vi "GyroTest.vi"() -> ()   [LabVIEW 2016]
uses:
  Gyro/GyroErrorCodes.ctl
  Telemetry/TelemetryFields.ctl
  <vilib>/rvi/Emulation/niFpgaGetClockAttributes.vi
  <vilib>/rvi/Emulation/niFpgaSctlEmulationGetInTimedLoop.vi
  <vilib>/rvi/Emulation/niFpgaEmulationReportErrorSimple.vi
  <vilib>/rvi/Emulation/niFpgaEmulationIsFPGAContextNoSignature.vi
  <vilib>/rvi/errors/niFpgaSetErrorForExecOnDevCompSimple.vi
  <vilib>/rvi/eio/common/nirviEmuReportErrorAndStop.vi
  <vilib>/rvi/DataTransferAndStorage/Container/Common/niFpgaContainerGetUniqueNameForEmu.vi
  <vilib>/rvi/FIFO/Fifo_Resource/nirvififoEmulationSetSize.vi
  <vilib>/rvi/FIFO/Fifo_Resource/nirviFifoEmulationQueueMgr.vi
  <instcachedir>/0/nirviFifoEmulationQueueMgr_E5CAEC123FF24DC58D834DCA3CDAA9B5.lvgen/nirviFifoEmulationQueueMgr_E5CAEC123FF24DC58D834DCA3CDAA9B5_004.vi
  <vilib>/Utility/error.llb/Clear Errors.vi
  <vilib>/rvi/FIFO/Fifo_Resource/nirvififoEmulationCreateLock.vi
  <vilib>/rvi/Emulation/niFpgaProcessEmulError.vi
  <vilib>/rvi/FIFO/Fifo_Resource/nirvififoEmulationObtainLock.vi
  <vilib>/rvi/FIFO/Fifo_Resource/nirvififoEmulationReleaseLock.vi
  <vilib>/rvi/occurrence/nirviWaitOnOccurrenceBase.vi
  <vilib>/rvi/errors/nirviReportUnexpectedCaseInternalError.vi
  <vilib>/rvi/errors/nirviReportUnexpectedCaseInternalError (U32).vi
  <vilib>/rvi/FIFO/Fifo_Resource/nirvififoEmulationDetermineInputValidOut.vi
  <vilib>/rvi/Emulation/niFpgaCriticalErrorInLSC.vi
  <instcachedir>/0/nirviFifoEmulationQueueMgr_E5CAEC123FF24DC58D834DCA3CDAA9B5.lvgen/nirviFifoEmulationQueueMgr_E5CAEC123FF24DC58D834DCA3CDAA9B5_028.vi
  <instcachedir>/0/nirviFifoEmulationQueueMgr_E5CAEC123FF24DC58D834DCA3CDAA9B5.lvgen/nirviFifoEmulationQueueMgr_E5CAEC123FF24DC58D834DCA3CDAA9B5_029.vi
  <instcachedir>/0/nirviFifoEmulationQueueMgr_E5CAEC123FF24DC58D834DCA3CDAA9B5.lvgen/nirviFifoEmulationQueueMgr_E5CAEC123FF24DC58D834DCA3CDAA9B5_039.vi
  <instcachedir>/0/nirviFifoEmulationQueueMgr_E5CAEC123FF24DC58D834DCA3CDAA9B5.lvgen/nirviFifoEmulationQueueMgr_E5CAEC123FF24DC58D834DCA3CDAA9B5_038.vi
  <instcachedir>/0/nirviFifoEmulationQueueMgr_E5CAEC123FF24DC58D834DCA3CDAA9B5.lvgen/nirviFifoEmulationQueueMgr_E5CAEC123FF24DC58D834DCA3CDAA9B5_035.vi
  <instcachedir>/0/nirviFifoEmulationQueueMgr_E5CAEC123FF24DC58D834DCA3CDAA9B5.lvgen/nirviFifoEmulationQueueMgr_E5CAEC123FF24DC58D834DCA3CDAA9B5_033.vi
  <instcachedir>/0/nirviFifoEmulationQueueMgr_E5CAEC123FF24DC58D834DCA3CDAA9B5.lvgen/nirviFifoEmulationQueueMgr_E5CAEC123FF24DC58D834DCA3CDAA9B5_009.vi
  <instcachedir>/0/nirviFifoEmulationQueueMgr_E5CAEC123FF24DC58D834DCA3CDAA9B5.lvgen/nirviFifoEmulationQueueMgr_E5CAEC123FF24DC58D834DCA3CDAA9B5_026.vi
  <vilib>/rvi/DataTransferAndStorage/Container/XNode/niFpgaContainer.xnode
  <vilib>/rvi/FIFO/Fifo_Resource/nirvififoEmulationRead.vi
  <vilib>/rvi/FIFO/Fifo_Resource/nirvififoEmulationWrite.vi
panel:
  out "GyroErrorCodeTimestamp":u64
  out "GyroErrorCode":T1
  out "GyroSampleTimestamp":u64
  out "GyroRxFrames":u64
  out "GyroTxFrames":u64
  out "GyroRxBytes":u64
  out "GyroTxBytes":u64
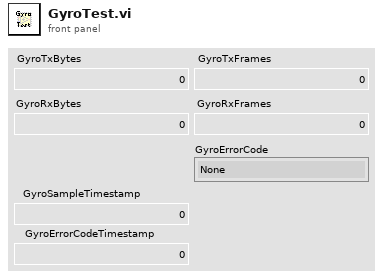
[diagram p1: front panel]
types:
  T1 = typedef "GyroErrorCodes.ctl" = enum8{"None", "ResponseHeaderError", "ResponseCRCError", "ResponseTimeoutError", "ResponseChecksumError"}
  T2 = cluster{"Timestamp":u64, "Accelerometer1Voltage":sgl, "Accelerometer2Voltage":sgl, "Accelerometer3Voltage":sgl, "Accelerometer4Voltage":sgl, "Accelerometer5Voltage":sgl, "Accelerometer6Voltage":sgl, "Accelerometer7Voltage":sgl, "Accelerometer8Voltage":sgl, "Accelerometer1Acceleration":sgl, "Accelerometer2Acceleration":sgl, "Accelerometer3Acceleration":sgl, "Accelerometer4Acceleration":sgl, "Accelerometer5Acceleration":sgl, "Accelerometer6Acceleration":sgl, "Accelerometer7Acceleration":sgl, "Accelerometer8Acceleration":sgl, "AngularAccelerationX":sgl, "AngularAccelerationY":sgl, "AngularAccelerationZ":sgl}
  T3 = cluster{"Timestamp":u64, "TxBytes":u64, "RxBytes":u64, "TxFrames":u64, "RxFrames":u64, "ErrorCode":enum8{"None", "ResponseAddressError", "ResponseFunctionCodeError", "ResponseByteCountError", "ResponseCRCError", "ResponseUnknownError", "ResponseTimeoutError", "SensorReportsIllegalFunction", "SensorReportsIllegalDataAddress"}}
  T4 = cluster{"Timestamp":u64, "TxBytes":u64, "RxBytes":u64, "TxFrames":u64, "RxFrames":u64, "RawAngle":i32, "ZenithAngle":sgl}
  T5 = cluster{"Timestamp":u64, "TxBytes":u64, "RxBytes":u64, "TxFrames":u64, "RxFrames":u64, "ErrorCode":enum16{"None", "ResponseUnknownError", "ResponseInvalidError", "ResponseTimeoutError", "SensorIndicatesInvalidCommandError", "SensorIndicatesCommunicationTimeoutError", "SensorIndicatesDataLengthError", "SensorIndicatesNumberOfParametersError", "SensorIndicatesParameterError", "SensorIndicatesCommunicationError", "SensorIndicatesIDNumberError", "SensorIndicatesExpansionLineError", "SensorIndicatesWriteControlError"}}
  T6 = cluster{"Timestamp":u64, "TxBytes":u64, "RxBytes":u64, "TxFrames":u64, "RxFrames":u64, "Sensor1Raw":i32, "Sensor2Raw":i32, "Sensor3Raw":i32, "Sensor4Raw":i32, "Sensor5Raw":i32, "Sensor6Raw":i32, "Sensor7Raw":i32, "Sensor8Raw":i32, "Sensor1Eng":sgl, "Sensor2Eng":sgl, "Sensor3Eng":sgl, "Sensor4Eng":sgl, "Sensor5Eng":sgl, "Sensor6Eng":sgl, "Sensor7Eng":sgl, "Sensor8Eng":sgl, "PositionX":sgl, "PositionY":sgl, "PositionZ":sgl, "RotationX":sgl, "RotationY":sgl, "RotationZ":sgl}
  T7 = typedef "TelemetryFields.ctl" = enum16{"None", "InclinometerTxBytes", "InclinometerRxBytes", "InclinometerTxFrames", "InclinometerRxFrames", "InclinometerErrorTimestamp", "InclinometerErrorCode", "InclinometerSampleTimestamp", "InclinometerRawAngle", "InclinometerZenithAngle", "DisplacementTxBytes", "DisplacementRxBytes", "DisplacementTxFrames", "DisplacementRxFrames", "DisplacementErrorTimestamp", "DisplacementErrorCode", "DisplacementSampleTimestamp", "DisplacementRaw1", "DisplacementRaw2", "DisplacementRaw3", "DisplacementRaw4", "DisplacementRaw5", "DisplacementRaw6", "DisplacementRaw7", "DisplacementRaw8", "DisplacementEng1", "DisplacementEng2", "DisplacementEng3", "DisplacementEng4", "DisplacementEng5", "DisplacementEng6", "DisplacementEng7", "DisplacementEng8", "DisplacementPositionX", "DisplacementPositionY", "DisplacementPositionZ", "DisplacementRotationX", "DisplacementRotationY", "DisplacementRotationZ", "AccelerometerSampleCount", "AccelerometerSampleTimestamp", "AccelerometerRaw1", "AccelerometerRaw2", "AccelerometerRaw3", "AccelerometerRaw4", "AccelerometerRaw5", "AccelerometerRaw6", "AccelerometerRaw7", "AccelerometerRaw8", "AccelerometerEng1", "AccelerometerEng2", "AccelerometerEng3", "AccelerometerEng4", "AccelerometerEng5", "AccelerometerEng6", "AccelerometerEng7", "AccelerometerEng8", "AngularAccelerationX", "AngularAccelerationY", "AngularAccelerationZ", "GyroTxBytes", "GyroRxBytes", "GyroTxFrames", "GyroRxFrames", "GyroErrorTimestamp", "GyroErrorCode", "GyroSampleTimestamp", "AngularVelocityX", "AngularVelocityY", "AngularVelocityZ", "GyroStatus", "GyroSequenceNumber", "GyroTemperature", "GyroBITTimestamp", "GyroBIT0", "GyroBIT1", "GyroBIT2", "GyroBIT3", "GyroBIT4", "GyroBIT5", "GyroBIT6", "GyroBIT7"}
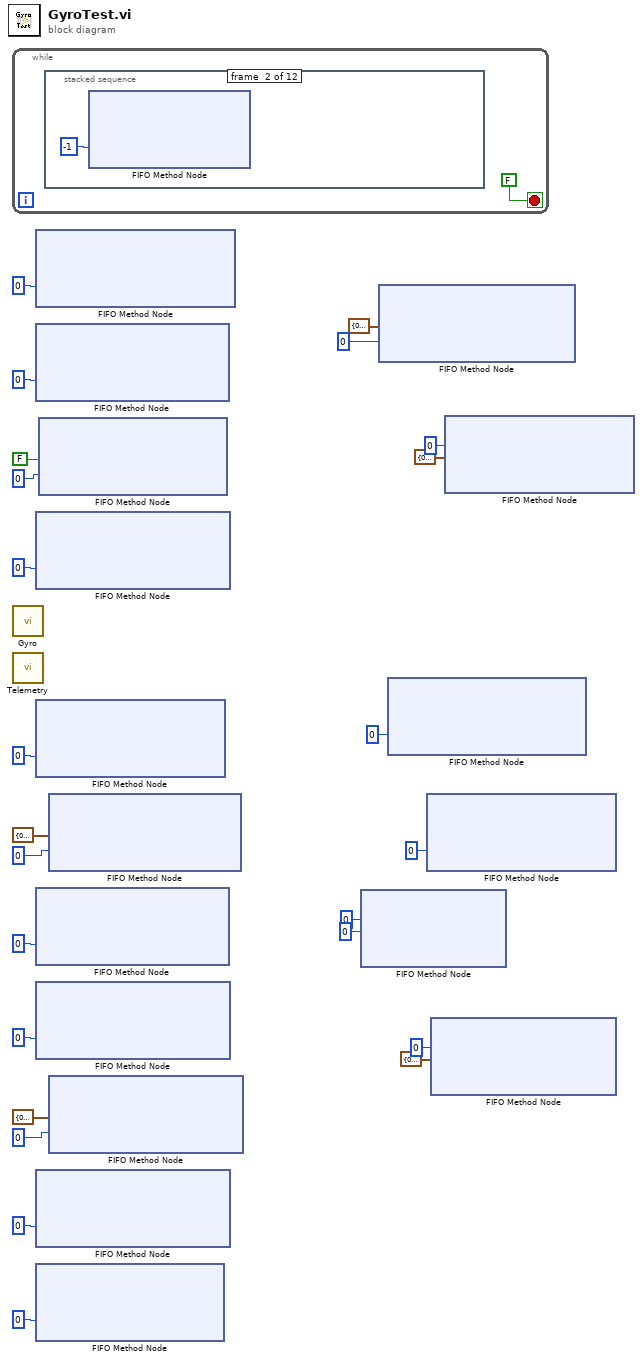
[diagram p0: block diagram]
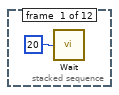
[diagram p2: hidden frame]
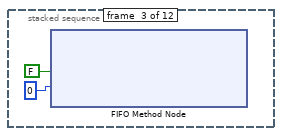
[diagram p3: hidden frame]
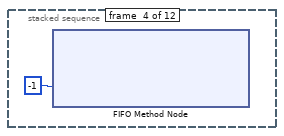
[diagram p4: hidden frame]
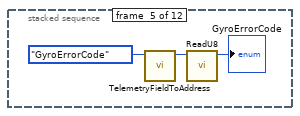
[diagram p5: hidden frame]
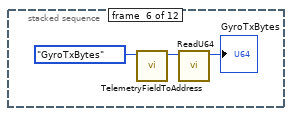
[diagram p6: hidden frame]
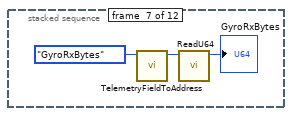
[diagram p7: hidden frame]
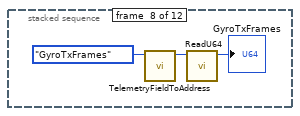
[diagram p8: hidden frame]
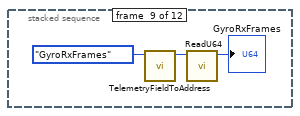
[diagram p9: hidden frame]
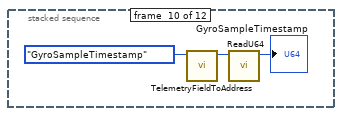
[diagram p10: hidden frame]
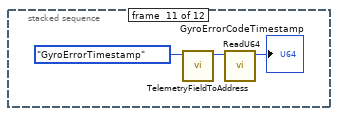
[diagram p11: hidden frame]
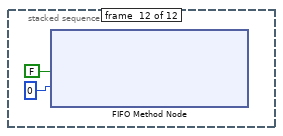
[diagram p12: hidden frame]
diagram:
  n1 = while {
    stop <- FALSE stop-if-true
    n2 = stacked-sequence {
      frame #0 {
        n3 = call "Wait"("Count(mSec)"=u32 20) -> ()  [unwired: 1 out]
      }
      frame #1 {
        n4 = xnode ("FIFO Method Node")("Timeout"=-1) -> ()  [unwired: 1 in, 3 out]
      }
      frame #2 {
        n5 = xnode ("FIFO Method Node")("Element"=FALSE, "Timeout"=0) -> ()  [unwired: 1 in, 2 out]
      }
      frame #3 {
        n6 = xnode ("FIFO Method Node")("Timeout"=-1) -> ()  [unwired: 1 in, 3 out]
      }
      frame #4 {
        n7 = call "TelemetryFieldToAddress.vi"("TelemetryFields"=TelemetryFields."GyroErrorCode") -> ("Address"=w33:u32)  [unwired: 10 in]
        n8 = call "ReadU8.vi"("Address"=w33) -> ("Data"=→"GyroErrorCode":u8)  [unwired: 10 in]
      }
      frame #5 {
        n9 = call "TelemetryFieldToAddress.vi"("TelemetryFields"=TelemetryFields."GyroTxBytes") -> ("Address"=w35:u32)  [unwired: 10 in]
        n10 = call "ReadU64.vi"("Address"=w35) -> ("Data"=→"GyroTxBytes":u64)  [unwired: 10 in]
      }
      frame #6 {
        n11 = call "TelemetryFieldToAddress.vi"("TelemetryFields"=TelemetryFields."GyroRxBytes") -> ("Address"=w38:u32)  [unwired: 10 in]
        n12 = call "ReadU64.vi"("Address"=w38) -> ("Data"=→"GyroRxBytes":u64)  [unwired: 10 in]
      }
      frame #7 {
        n13 = call "TelemetryFieldToAddress.vi"("TelemetryFields"=TelemetryFields."GyroTxFrames") -> ("Address"=w41:u32)  [unwired: 10 in]
        n14 = call "ReadU64.vi"("Address"=w41) -> ("Data"=→"GyroTxFrames":u64)  [unwired: 10 in]
      }
      frame #8 {
        n15 = call "TelemetryFieldToAddress.vi"("TelemetryFields"=TelemetryFields."GyroRxFrames") -> ("Address"=w44:u32)  [unwired: 10 in]
        n16 = call "ReadU64.vi"("Address"=w44) -> ("Data"=→"GyroRxFrames":u64)  [unwired: 10 in]
      }
      frame #9 {
        n17 = call "TelemetryFieldToAddress.vi"("TelemetryFields"=TelemetryFields."GyroSampleTimestamp") -> ("Address"=w47:u32)  [unwired: 10 in]
        n18 = call "ReadU64.vi"("Address"=w47) -> ("Data"=→"GyroSampleTimestamp":u64)  [unwired: 10 in]
      }
      frame #10 {
        n19 = call "TelemetryFieldToAddress.vi"("TelemetryFields"=TelemetryFields."GyroErrorTimestamp") -> ("Address"=w50:u32)  [unwired: 10 in]
        n20 = call "ReadU64.vi"("Address"=w50) -> ("Data"=→"GyroErrorCodeTimestamp":u64)  [unwired: 10 in]
      }
      frame #11 {
        n21 = xnode ("FIFO Method Node")("Element"=FALSE, "Timeout"=0) -> ()  [unwired: 1 in, 2 out]
      }
    }
  }
  n22 = call "Gyro.vi"() -> ()  [unwired: 12 in]
  n23 = call "Telemetry.vi"() -> ()  [unwired: 12 in]
  n24 = xnode ("FIFO Method Node")("Timeout"=0) -> ()  [unwired: 1 in, 3 out]
  n25 = xnode ("FIFO Method Node")("Timeout"=0) -> ()  [unwired: 1 in, 3 out]
  n26 = xnode ("FIFO Method Node")("Timeout"=0) -> ()  [unwired: 1 in, 3 out]
  n27 = xnode ("FIFO Method Node")("Timeout"=0) -> ()  [unwired: 1 in, 3 out]
  n28 = xnode ("FIFO Method Node")("Timeout"=0) -> ()  [unwired: 1 in, 3 out]
  n29 = xnode ("FIFO Method Node")("Timeout"=0) -> ()  [unwired: 1 in, 3 out]
  n30 = xnode ("FIFO Method Node")("Timeout"=0) -> ()  [unwired: 1 in, 3 out]
  n31 = xnode ("FIFO Method Node")("Timeout"=0) -> ()  [unwired: 1 in, 3 out]
  n32 = xnode ("FIFO Method Node")("Element"=FALSE, "Timeout"=0) -> ()  [unwired: 1 in, 2 out]
  n33 = xnode ("FIFO Method Node")("Element"=T6 {"Timestamp"=0, "TxBytes"=0, "RxBytes"=0, "TxFrames"=0, "RxFrames"=0, "Sensor1Raw"=0, "Sensor2Raw"=0, "Sensor3Raw"=0, "Sensor4Raw"=0, "Sensor5Raw"=0, "Sensor6Raw"=0, "Sensor7Raw"=0, "Sensor8Raw"=0, "Sensor1Eng"=0.0, "Sensor2Eng"=0.0, "Sensor3Eng"=0.0, "Sensor4Eng"=0.0, "Sensor5Eng"=0.0, "Sensor6Eng"=0.0, "Sensor7Eng"=0.0, "Sensor8Eng"=0.0, "PositionX"=0.0, "PositionY"=0.0, "PositionZ"=0.0, "RotationX"=0.0, "RotationY"=0.0, "RotationZ"=0.0}, "Timeout"=0) -> ()  [unwired: 1 in, 2 out]
  n34 = xnode ("FIFO Method Node")("Element"=T5 {"Timestamp"=0, "TxBytes"=0, "RxBytes"=0, "TxFrames"=0, "RxFrames"=0, "ErrorCode"=enum."None"}, "Timeout"=0) -> ()  [unwired: 1 in, 2 out]
  n35 = xnode ("FIFO Method Node")("Element"=u8 0, "Timeout"=0) -> ()  [unwired: 1 in, 2 out]
  n36 = xnode ("FIFO Method Node")("Element"=T4 {"Timestamp"=0, "TxBytes"=0, "RxBytes"=0, "TxFrames"=0, "RxFrames"=0, "RawAngle"=0, "ZenithAngle"=0.0}, "Timeout"=0) -> ()  [unwired: 1 in, 2 out]
  n37 = xnode ("FIFO Method Node")("Timeout"=0) -> ()  [unwired: 1 in, 3 out]
  n38 = xnode ("FIFO Method Node")("Timeout"=0) -> ()  [unwired: 1 in, 3 out]
  n39 = xnode ("FIFO Method Node")("Element"=T2 {"Timestamp"=0, "Accelerometer1Voltage"=0.0, "Accelerometer2Voltage"=0.0, "Accelerometer3Voltage"=0.0, "Accelerometer4Voltage"=0.0, "Accelerometer5Voltage"=0.0, "Accelerometer6Voltage"=0.0, "Accelerometer7Voltage"=0.0, "Accelerometer8Voltage"=0.0, "Accelerometer1Acceleration"=0.0, "Accelerometer2Acceleration"=0.0, "Accelerometer3Acceleration"=0.0, "Accelerometer4Acceleration"=0.0, "Accelerometer5Acceleration"=0.0, "Accelerometer6Acceleration"=0.0, "Accelerometer7Acceleration"=0.0, "Accelerometer8Acceleration"=0.0, "AngularAccelerationX"=0.0, "AngularAccelerationY"=0.0, "AngularAccelerationZ"=0.0}, "Timeout"=0) -> ()  [unwired: 1 in, 2 out]
  n40 = xnode ("FIFO Method Node")("Element"=T3 {"Timestamp"=0, "TxBytes"=0, "RxBytes"=0, "TxFrames"=0, "RxFrames"=0, "ErrorCode"=enum."None"}, "Timeout"=0) -> ()  [unwired: 1 in, 2 out]
